vi "rad_Get Backplane Type.vi"(8 "error in (no error)":errorcluster, 11 "Controller IP":string) -> (0 "error out":errorcluster, 2 "Backplane Type":string, 3 "Controller IP Out":string)   [LabVIEW 2013]
panel:
  out "cRIO Backplane":T1(ring)
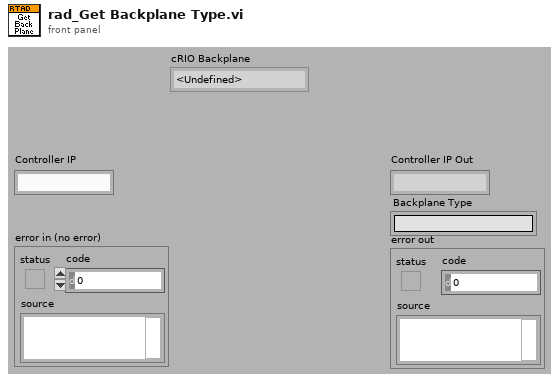
[diagram p1: front panel]
types:
  T1 = enum16{"<Undefined>", "cRIO-9101", "cRIO-9102", "cRIO-9103", "cRIO-9104", "cRIO-9072", "cRIO-9074"}
  T2 = typedef "cri_cRIO Backplane Info.ctl" = cluster{"Model Name":string, "Model Code":u32, "Serial Number":u32, "cRIO Backplane":T3}
  T3 = typedef "cri_cRIO Backplanes.ctl" = enum16{"<Undefined>", "cRIO-9101", "cRIO-9102", "cRIO-9103", "cRIO-9104", "cRIO-9072", "cRIO-9074"}
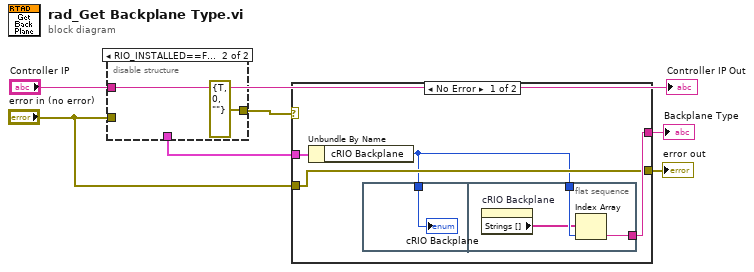
[diagram p0: block diagram]
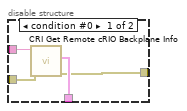
[diagram p2: hidden frame]
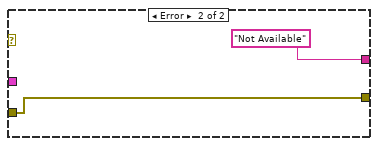
[diagram p3: hidden frame]
diagram:
  n1 = disable-structure shown="RIO_INSTALLED==False, default" {
    disable-tunnel: "Controller IP" -> [w10 _]
    disable-tunnel: [w9 _] -> w5
    disable-tunnel: [w8 errorcluster {"status"=TRUE, "code"=0, "source"=""} ("error out")] -> w4
    disable-tunnel: "error in (no error)" -> [w7 _]
    frame condition #0 {
      n2 = call <userlib>:"CRI Get Remote cRIO Backplane Info.vi"("error in (no error)"=w7, "IP Address"=w10) -> ("error out"=w8:errorcluster, "cRIO Backplane Information"=w9:T2)  [unwired: 8 in]
    }
    frame condition #1 (active) {
    }
  }
  n3 = case shown="No Error" w4 {
    tunnel: w5 -> [w15 _]
    tunnel: [w14 "Not Available"] -> w2
    tunnel: [w13 w21] -> w1
    tunnel: "error in (no error)" -> [w13 w21]
    frame No Error {
      n4 = Unbundle By Name(w15) -> ("cRIO Backplane"=w12:T3)
      n5 = flat-sequence {
        tunnel: w12 -> [w16]
        tunnel: w12 -> [w19]
        tunnel: [w18] -> w14
        frame #0 {
          "cRIO Backplane" <- w16
        }
        frame #1 {
          n6 = property on="cRIO Backplane" class="Enum (strict)"() -> ("Strings []"=w17:string[])  [unwired: 2 in, 2 out]
          n7 = Index Array(array=w17, index=w19) -> (element=w18:string)
        }
      }
    }
    frame Error {
    }
  }
  "Backplane Type" <- w2
  "error out" <- w1
  "Controller IP Out" <- "Controller IP"
